vi "odor config arr to disabled odors array (sub-vi).vi"(10 "odor descriptions":T1) -> (2 "Disabled Items []":i32[](array[numeric]))   [LabVIEW 2021]
uses:
  type-defs/odor description array (type def).ctl
  type-defs/odor info cluster (type def).ctl
  type-defs/odor selection (type def).ctl
  type-defs/odor color (type def).ctl
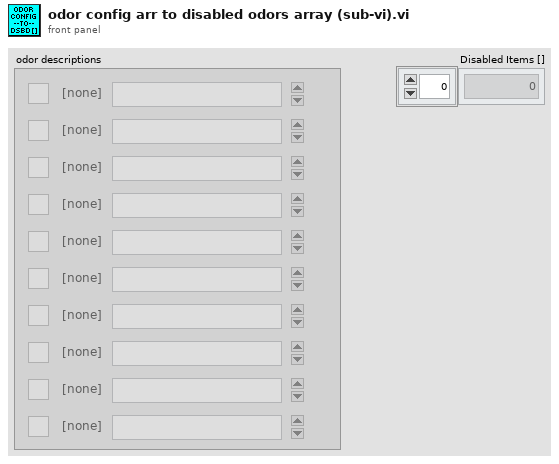
[diagram p1: front panel]
types:
  T1 = typedef "odor description array (type def).ctl" = T2[]
  T2 = typedef "odor info cluster (type def).ctl" = cluster{"odor channel":T3, "odor description":string, "odor color":T4, "odor channel active":bool}
  T3 = typedef "odor selection (type def).ctl" = enum16{"[none]", "odor 1", "odor 2", "odor 3", "odor 4", "odor 5", "odor 6", "odor 7", "odor 8", "odor 9", "odor 10"}
  T4 = typedef "odor color (type def).ctl" = u16
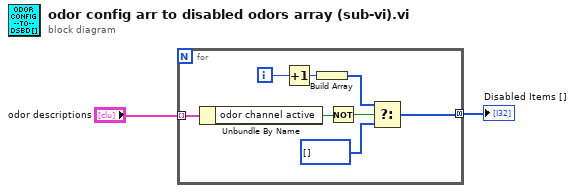
[diagram p0: block diagram]
diagram:
  n1 = for {
    tunnel: "odor descriptions" -> [w10] mode=indexing
    tunnel: [w4] -> w2 mode=concatenating
    i -> [w7]
    n2 = Unbundle By Name(w10) -> ("odor channel active"=w9:bool)
    n3 = Increment(x=w7) -> (x+1=w3:i32)
    n4 = Build Array(w3) -> (w5:i32[])
    n5 = Not(x=w9) -> (.not. x?=w8:bool)
    n6 = Select(t=w5, s=w8, f=i32[] [] ("Disabled Items []")) -> (s? t:f=w4:i32[])
  }
  "Disabled Items []" <- w2
